vi "Stage Labview control.vi"() -> ()   [LabVIEW 2020]
uses:
  <vilib>/DAQmx/write.llb/DAQmx Write (Analog 1D Wfm NChan NSamp).vi
  <vilib>/DAQmx/create/channels.llb/DAQmx Create Channel (AO-Voltage-Basic).vi
  <vilib>/Analysis/1siggen.llb/Ramp Pattern by Delta.vi
  <vilib>/DAQmx/configure/timing.llb/DAQmx Timing (Use Waveform).vi
  <vilib>/DAQmx/miscellaneous.llb/DAQmx Fill In Error Info.vi
  <vilib>/Analysis/NI_AALBase.lvlib
panel:
  in  "Enable z axis":bool
  in  "FPosition":dbl
  out "Ramp Graph":dbl[](graph)
  out "x*y=Tot Z thickness/(Z slice width* # of slices)":dbl
  out "Waveform Graph":waveform(dbl)[](graph)
  out "Square wave Graph":dbl[](graph)
  out "Sawtooth Graph":dbl[](graph)
  out "AO (number of samples written per channel)":u32
  out "Number of slices":dbl
  in  "End position (mm)":dbl
  out "Total Z thickness (mm)":dbl
  in  "Z slice width (mm)":dbl
  in  "Start position(mm)":dbl
  in  "Z stack?":bool
  in  "Disable all Axes?":bool
  out "Z Position":dbl
  out "Error out":errorcluster
  out "Z Position":dbl
  out "Connected":bool
  out "GetFirmwareVersion 2":string
  in  "SPIIPLUSCOM660Lib.IAsyncChannel":refnum<k7>
  # "100um"
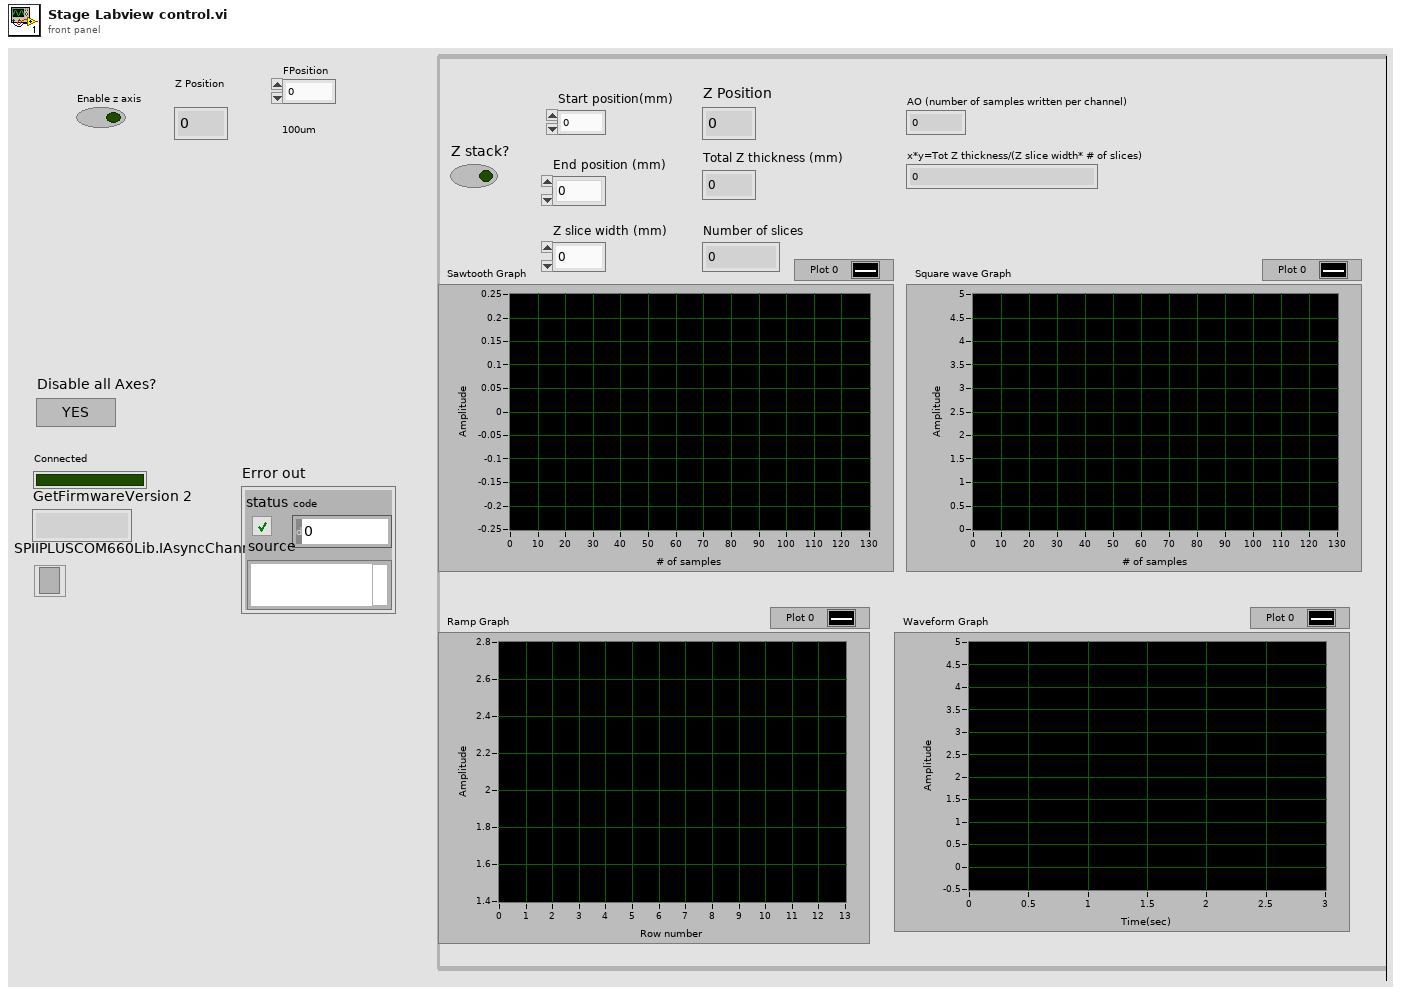
[diagram p1: front panel]
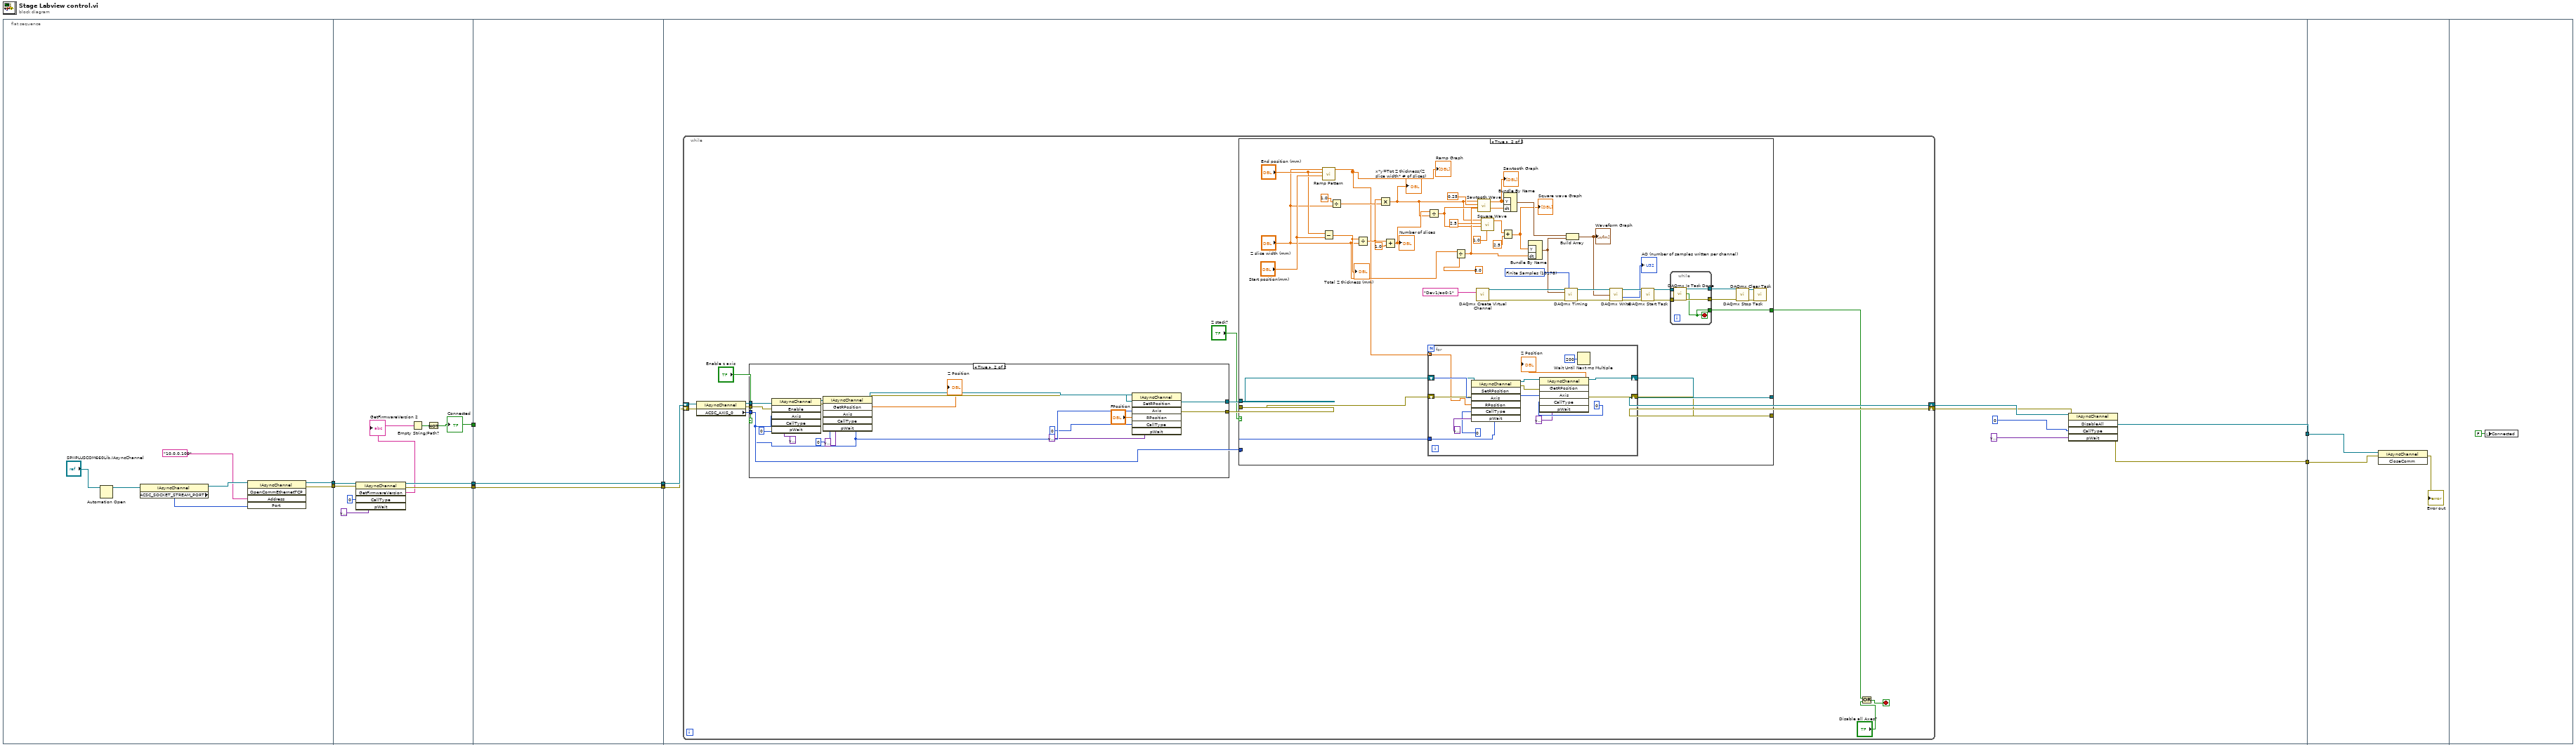
[diagram p0: block diagram]
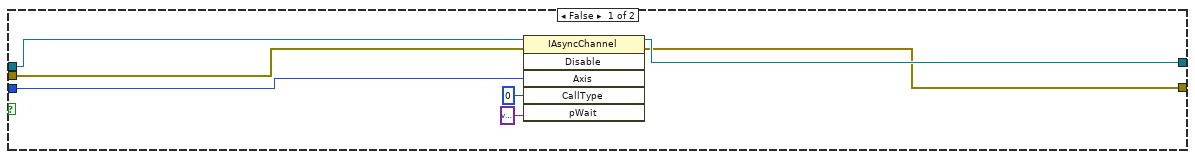
[diagram p2: hidden frame]
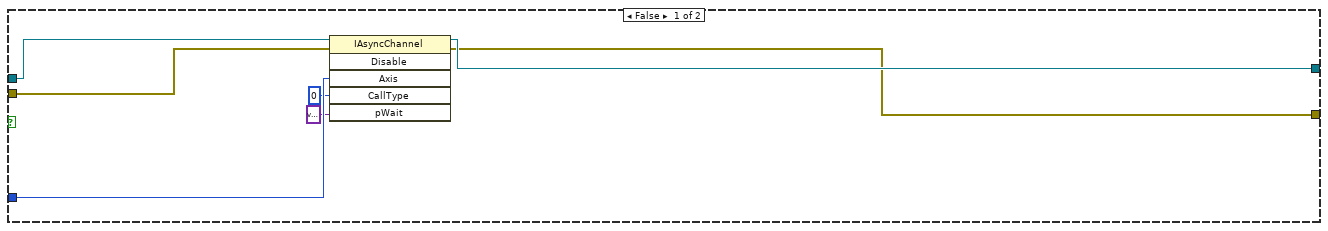
[diagram p3: hidden frame]
diagram:
  n1 = flat-sequence {
    tunnel: [w12] -> w9
    tunnel: [w11] -> w8
    tunnel: w9 -> [w25]
    tunnel: w8 -> [w22]
    tunnel: [w21] -> w7
    tunnel: [w20] -> w6
    tunnel: [w17] -> w5
    tunnel: w7 -> [w26]
    tunnel: w6 -> [w27]
    tunnel: w5 -> [_]
    tunnel: [w27] -> w4
    tunnel: [w26] -> w2
    tunnel: w4 -> [w31]
    tunnel: [w33] -> w3
    tunnel: w2 -> [w30]
    tunnel: [w32] -> w1
    tunnel: w3 -> [w147]
    tunnel: w1 -> [w146]
    frame #0 {
      n2 = Automation Open(Automation Refnum="SPIIPLUSCOM660Lib.IAsyncChannel") -> (Automation Refnum=w16:refnum<k7>)  [unwired: 3 in, 1 out]
      n3 = property class="IAsyncChannel"(reference=w16) -> (reference out=w15:refnum<k7>, "ACSC_SOCKET_STREAM_PORT"=w13:i32)  [unwired: 1 in, 1 out]
      n4 = invoke class="IAsyncChannel" method="OpenCommEthernetTCP"(reference=w15, "Address"="10.0.0.100", "Port"=w13) -> (reference out=w12:refnum<k7>, error out=w11:errorcluster)  [unwired: 2 in, 3 out]
    }
    frame #1 {
      n5 = invoke class="IAsyncChannel" method="GetFirmwareVersion"(reference=w25, error in=w22, "CallType"=u64 0, "pWait"=variant) -> (reference out=w20:refnum<k7>, error out=w21:errorcluster, "GetFirmwareVersion"=w19:string)  [unwired: 1 in, 2 out]
      "GetFirmwareVersion 2" <- w19
      n6 = Empty String/Path?(string/path=w19) -> (empty?=w18:bool)
      n7 = Not(x=w18) -> (.not. x?=w17:bool)
      "Connected" <- w17
    }
    frame #2 {
    }
    frame #3 {
      n8 = while {
        shift-right: [w47] -> w35
        shift-left: w31 -> [w49]
        shift-right: [w46] -> w34
        shift-left: w30 -> [w48]
        stop <- w39 stop-if-true
        n9 = property class="IAsyncChannel"(reference=w49, error in=w48) -> (reference out=w45:refnum<k7>, error out=w42:errorcluster, "ACSC_AXIS_0"=w41:i32)
        n10 = case shown="True" "Enable z axis" {
          tunnel: w45 -> [w56 w73]
          tunnel: [w54 w72] -> w44
          tunnel: [w53 w71] -> w43
          tunnel: w42 -> [w55 w70]
          tunnel: w41 -> [w52 w69]
          frame False {
            n11 = invoke class="IAsyncChannel" method="Disable"(reference=w56, error in=w55, "Axis"=w52, "CallType"=u64 0, "pWait"=variant) -> (reference out=w54:refnum<k7>, error out=w53:errorcluster)  [unwired: 1 in, 4 out]
          }
          frame True {
            n12 = invoke class="IAsyncChannel" method="Enable"(reference=w73, error in=w70, "Axis"=w69, "CallType"=u64 0, "pWait"=variant) -> (reference out=w66:refnum<k7>, error out=w65:errorcluster)  [unwired: 1 in, 4 out]
            n13 = invoke class="IAsyncChannel" method="GetRPosition"(reference=w66, error in=w65, "Axis"=w69, "CallType"=u64 0, "pWait"=variant) -> (reference out=w64:refnum<k7>, error out=w61:errorcluster, "GetRPosition"=→"Z Position":dbl)  [unwired: 1 in, 3 out]
            n14 = invoke class="IAsyncChannel" method="SetRPosition"(reference=w64, error in=w61, "Axis"=w69, "RPosition"="FPosition", "CallType"=u64 0, "pWait"=variant) -> (reference out=w72:refnum<k7>, error out=w71:errorcluster)  [unwired: 1 in, 5 out]
          }
        }
        n15 = case shown="True" "Z stack?" {
          tunnel: [w75 w125] -> w47
          tunnel: [w74 w124] -> w46
          tunnel: w44 -> [w80 w121]
          tunnel: w43 -> [w79 w123]
          tunnel: w41 -> [w78 w122]
          tunnel: [_ w84] -> w38
          frame False {
            n16 = invoke class="IAsyncChannel" method="Disable"(reference=w80, error in=w79, "Axis"=w78, "CallType"=u64 0, "pWait"=variant) -> (reference out=w75:refnum<k7>, error out=w74:errorcluster)  [unwired: 1 in, 4 out]
          }
          frame True {
            w115 = 10178 items=["Finite Samples"=10178, "Continuous Samples"=10123, "Hardware Timed Single Point"=12522] ("sample mode")
            n17 = call-poly <vilib>:"Ramp Pattern.vi"("start"="Start position(mm)", "end"="End position (mm)", "delta"="Z slice width (mm)") -> ("Ramp Pattern"=w85:dbl[])  [unwired: 6 in, 2 out]
            "Ramp Graph" <- w85
            n18 = Subtract(x="End position (mm)", y="Start position(mm)") -> (x-y=w105:dbl)
            "Total Z thickness (mm)" <- w105
            n19 = Divide(x=1.0, y="Z slice width (mm)") -> (x/y=w91:dbl)
            n20 = Divide(x=w105, y="Z slice width (mm)") -> (x/y=w95:dbl)
            n21 = Multiply(x=w95, y=w91) -> (x*y=w90:dbl)
            "x*y=Tot Z thickness/(Z slice width* # of slices)" <- w90
            n22 = Add(x=w95, y=1.0) -> (x+y=w97:dbl)
            "Number of slices" <- w97
            n23 = Divide(x=w97, y=w90) -> (x/y=w96:dbl)
            n24 = for {
              tunnel: w122 -> [w142]
              shift-right: [w144] -> w125
              shift-left: w121 -> [w139]
              shift-right: [w143] -> w124
              shift-left: w123 -> [w138]
              tunnel: w85 -> [w132] mode=indexing
              n25 = invoke class="IAsyncChannel" method="SetRPosition"(reference=w139, error in=w138, "Axis"=w142, "RPosition"=w132, "CallType"=u64 0, "pWait"=variant) -> (reference out=w137:refnum<k7>, error out=w136:errorcluster)  [unwired: 1 in, 5 out]
              n26 = invoke class="IAsyncChannel" method="GetRPosition"(reference=w137, error in=w136, "Axis"=w142, "CallType"=u64 0, "pWait"=variant) -> (reference out=w144:refnum<k7>, error out=w143:errorcluster, "GetRPosition"=→"Z Position":dbl)  [unwired: 1 in, 3 out]
              n27 = Wait Until Next ms Multiple(millisecond multiple=u32 200) -> ()  [unwired: 1 out]
            }
            n28 = Divide(x="Z slice width (mm)", y=5.0) -> (x/y=w98:dbl)
            n29 = call-poly <vilib>:"DAQmx Create Virtual Channel.vi"("physical channels"=tag "Dev1/ao0:1") -> ("task out"=w120:refnum<k21>, "error out"=w119:errorcluster)  [unwired: 13 in]
            n30 = call <vilib>:"Sawtooth Wave.vi"("samples"=w90, "amplitude"=0.25, "frequency"=w96) -> ("sawtooth wave"=w100:dbl[])  [unwired: 2 in, 2 out]
            "Sawtooth Graph" <- w100
            n31 = call <vilib>:"Square Wave.vi"("samples"=w90, "amplitude"=2.5, "frequency"=w96, "duty cycle (%)"=1.0) -> ("square wave"=w82:dbl[])  [unwired: 2 in, 2 out]
            n32 = Add(x=w82, y=2.5) -> (x+y=w81:dbl[])
            "Square wave Graph" <- w81
            n33 = Bundle By Name("Y"=w100, "dt"=w98) -> (w106:waveform(dbl))  [unwired: 1 in]
            n34 = Bundle By Name("Y"=w81, "dt"=w98) -> (w94:waveform(dbl))  [unwired: 1 in]
            n35 = call-poly <vilib>:"DAQmx Timing.vi"("task/channels in"=w120, "sample mode"=w115, "waveform"=w94, "error in"=w119) -> ("task out"=w113:refnum<k21>, "error out"=w110:errorcluster)  [unwired: 10 in]
            n36 = Build Array(w106, w94) -> (w99:waveform(dbl)[])
            "Waveform Graph" <- w99
            n37 = call-poly <vilib>:"DAQmx Write.vi"("task/channels in"=w113, "data"=w99, "error in"=w110) -> ("task out"=w109:refnum<k21>, "number of samples written per channel"=→"AO (number of samples written per channel)":u32, "error out"=w108:errorcluster)  [unwired: 10 in]
            n38 = call <vilib>:"DAQmx Start Task.vi"("task/channels in"=w109, "error in"=w108) -> ("task out"=w89:refnum<k21>, "error out"=w88:errorcluster)  [unwired: 12 in]
            n39 = while {
              tunnel: w89 -> [w130]
              tunnel: w88 -> [w129]
              tunnel: [w128] -> w87
              tunnel: [w127] -> w86
              tunnel: [w126] -> w84
              stop <- w126 stop-if-true
              n40 = call <vilib>:"DAQmx Is Task Done.vi"("task/channels in"=w130, "error in"=w129) -> ("task out"=w128:refnum<k21>, "task done?"=w126:bool, "error out"=w127:errorcluster)  [unwired: 11 in]
            }
            n41 = call <vilib>:"DAQmx Stop Task.vi"("task/channels in"=w87, "error in"=w86) -> ("task out"=w117:refnum<k21>, "error out"=w116:errorcluster)  [unwired: 12 in]
            n42 = call <vilib>:"DAQmx Clear Task.vi"("task in"=w117, "error in"=w116) -> ()  [unwired: 13 in, 1 out]
          }
        }
        n43 = Or(x=w38, y="Disable all Axes?") -> (x .or. y?=w39:bool)
      }
      n44 = invoke class="IAsyncChannel" method="DisableAll"(reference=w35, error in=w34, "CallType"=u64 0, "pWait"=variant) -> (reference out=w33:refnum<k7>, error out=w32:errorcluster)  [unwired: 1 in, 3 out]
    }
    frame #4 {
      n45 = invoke class="IAsyncChannel" method="CloseComm"(reference=w147, error in=w146) -> (error out=→"Error out":errorcluster)  [unwired: 1 in, 2 out]
    }
    frame #5 {
      n46 = local write "Connected"(FALSE ("Connected")) -> ()
    }
  }
